vi "mergeFractionalSeconds.vi"(9 "Fractional Second":dbl format="%#.6f", 10 "(Integer) Time (s)":i64, 11 "Epoch in":refnum<class "Epoch.lvclass">) -> (2 "(Float) Time (s)":dbl format="%#.6f", 3 "Epoch out":refnum<class "Epoch.lvclass">)   [LabVIEW 2013, in "Epoch.lvclass"]
uses:
  Epoch.lvclass
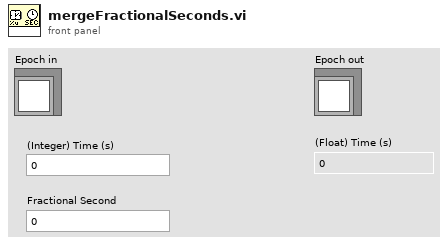
[diagram p1: front panel]
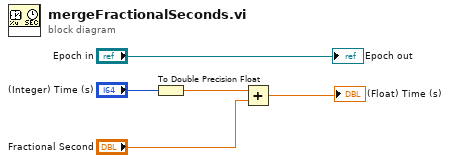
[diagram p0: block diagram]
diagram:
  n1 = To Double Precision Float(number="(Integer) Time (s)") -> (double precision float=w1:dbl)
  n2 = Add(x=w1, y="Fractional Second") -> (x+y=→"(Float) Time (s)":dbl)
  "Epoch out" <- "Epoch in"
